vi "CommonVIs_Wait.vi"(9 "error in":errorcluster, 10 "Wait(150ms)":u32=150) -> (2 "error out":errorcluster)   [LabVIEW 2012]
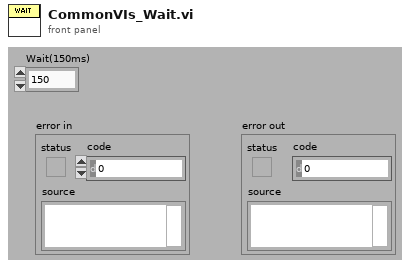
[diagram p1: front panel]
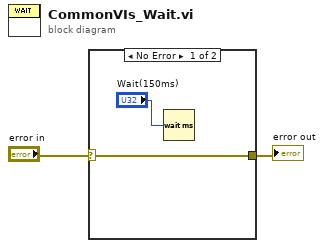
[diagram p0: block diagram]
diagram:
  n1 = case shown="No Error" "error in" {
    selector: "error in" -> [w3 w5]
    tunnel: [w3 w5] -> w1
    frame No Error {
      n2 = Wait (ms)(milliseconds to wait="Wait(150ms)") -> ()  [unwired: 1 out]
    }
    frame Error {
    }
  }
  "error out" <- w1
